vi "Lookup Response Info.vi"(8 "error in (no error)":errorcluster, 9 "Wait Value Channel Lookup Info":T6 {"Refs" format="%.0x"}, 10 "Resp Channel Lookup Info":T6 {"Refs" format="%.0x"}, 11 "Section Ref in":T1 format="%.0x") -> (0 "error out":errorcluster, 1 "Wait Value Channel Lookup Info out":T6 {"Refs" format="%.0x"}, 2 "Resp Channel Lookup Info out":T6 {"Refs" format="%.0x"}, 3 "Section Ref out":T1 format="%.0x", 5 "Response Info":T2)   [LabVIEW 2018, in "Instrument Addon System Explorer.lvlib"]
uses:
  Instrument Addon System Explorer.lvlib
  <vilib>/NI VeriStand/Custom Device Tools/Custom Device Utility Library/Custom Device Utility Library.lvlib
  <vilib>/NI VeriStand/Custom Device Tools/Custom Device Utility Library/NI VeriStand - Search for Item by GUID.vi
  Addon Shared/SubVIs/Constants.vi
  Addon Shared/Instrument Addon Shared.lvlib
  Addon Shared/Types/Response Wait Type.ctl
  Addon Shared/Types/Linked Channel Cluster.ctl
  Addon Shared/Types/Response Parameters.ctl
  Addon Shared/Types/Response RT Configuration Cluster.ctl
  Addon Shared/Types/FG Control.ctl
  <vilib>/NI VeriStand/Custom Device API/Custom Device API.lvlib
  <vilib>/NI VeriStand/Custom Device API/Custom Device Item Ref.ctl
  Types/Channel Lookup Cluster.ctl
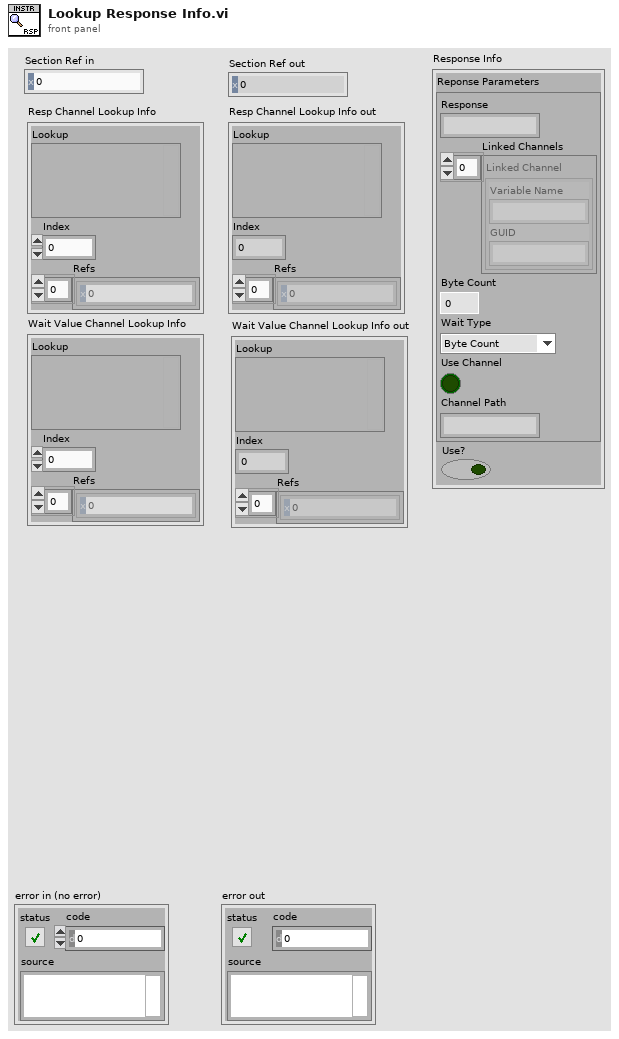
[diagram p1: front panel]
types:
  T1 = typedef "Custom Device API.lvlib/Custom Device Item Ref.ctl" = u64
  T2 = typedef "Instrument Addon Shared.lvlib/Response RT Configuration Cluster.ctl" = cluster{"Reponse Parameters":T3, "Use?":bool}
  T3 = typedef "Instrument Addon Shared.lvlib/Response Parameters.ctl" = cluster{"Response":string, "Linked Channels":T4[], "Type Value":dbl, "Wait Type":T5, "Use Channel":bool, "Channel Path":string}
  T4 = typedef "Instrument Addon Shared.lvlib/Linked Channel Cluster.ctl" = cluster{"Variable Name":string, "GUID":string}
  T5 = typedef "Instrument Addon Shared.lvlib/Response Wait Type.ctl" = enum16{"Byte Count", "Wait sec"}
  T6 = typedef "Instrument Addon System Explorer.lvlib/Channel Lookup Cluster.ctl" = cluster{"Lookup":variant, "Index":i32, "Refs":T1[]}
  T7 = typedef "Instrument Addon Shared.lvlib/FG Control.ctl" = enum16{"Get", "Set"}
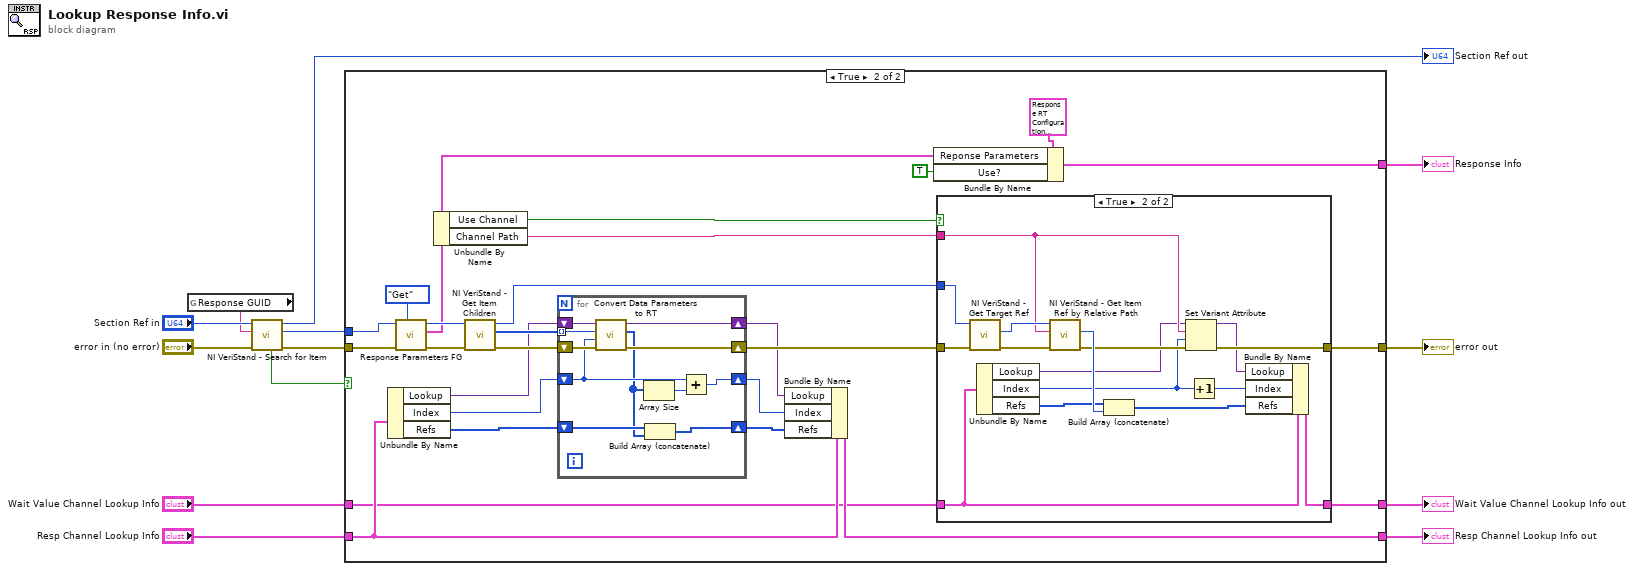
[diagram p0: block diagram]
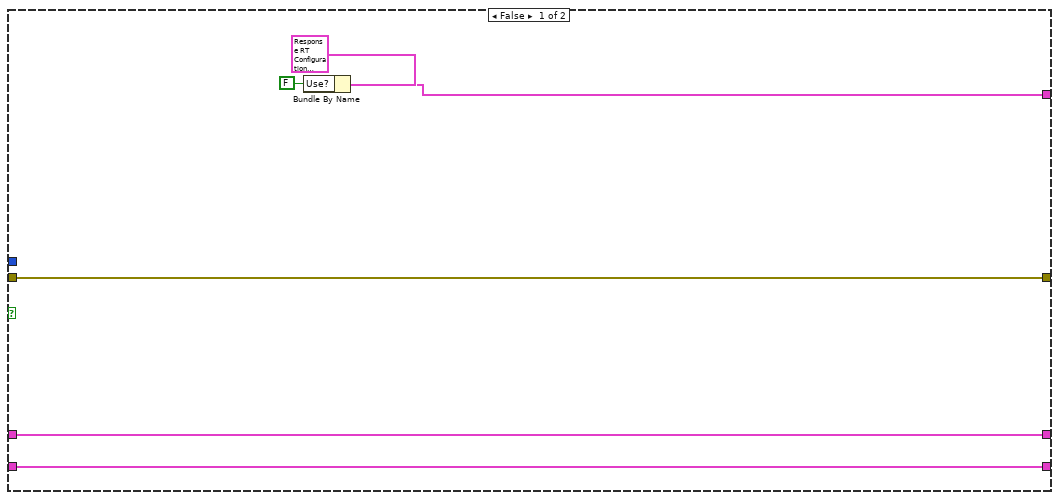
[diagram p2: hidden frame]
diagram:
  n1 = global read "Constants.vi" "Response GUID"() -> (w6:string)
  n2 = call-poly <vilib>:"NI VeriStand - Search for Item.vi"("error in"="error in (no error)", "Item GUID"=w6, "Section Ref in"="Section Ref in") -> ("error out"=w9:errorcluster, "Item Ref"=w10:T1, "Section Ref out"=→"Section Ref out":T1, "Found"=w13:bool)  [unwired: 5 in]
  n3 = case shown="True" w13 {
    tunnel: w9 -> [w19 w44]
    tunnel: w10 -> [_ w43]
    tunnel: [w17 w39] -> w11
    tunnel: [w19 w33] -> w12
    tunnel: "Resp Channel Lookup Info" -> [w15 w27]
    tunnel: [w15 w26] -> w4
    tunnel: "Wait Value Channel Lookup Info" -> [w14 w25]
    tunnel: [w14 w24] -> w2
    frame False {
      n4 = Bundle By Name(cluster=T2 {"Reponse Parameters"={"Response"="", "Linked Channels"=[], "Type Value"=0.0, "Wait Type"=enum."Byte Count", "Use Channel"=FALSE, "Channel Path"=""}, "Use?"=FALSE}, "Use?"=FALSE) -> (w17:T2)
    }
    frame True {
      n5 = Unbundle By Name(w27) -> ("Lookup"=w31:variant, "Index"=w30:i32, "Refs"=w21:T1[])
      n6 = call "Response Parameters FG.vi"("Action"=FG_Control."Get", "error in (no error)"=w44, "Item Ref in"=w43) -> ("error out"=w36:errorcluster, "Reponse Parameters"=w37:T3, "Item Ref out"=w42:T1)  [unwired: 6 in]
      n7 = Unbundle By Name(w37) -> ("Use Channel"=w22:bool, "Channel Path"=w35:string)
      n8 = call <vilib>:"NI VeriStand - Get Item Children.vi"("error in (no error)"=w36, "Item Ref in"=w42) -> ("error out"=w41:errorcluster, "Child Refs"=w38:T1[], "Item Ref out"=w32:T1)  [unwired: 6 in, 1 out]
      n9 = for {
        shift-right: [w71] -> w34
        shift-left: w41 -> [w74]
        tunnel: w38 -> [w73] mode=indexing
        shift-right: [w64] -> w29
        shift-left: w30 -> [w66]
        shift-right: [w70] -> w28
        shift-left: w31 -> [w72]
        shift-right: [w68] -> w20
        shift-left: w21 -> [w69]
        n10 = call "Convert Data Parameters to RT.vi"("error in (no error)"=w74, "Data Index"=w66, "Item Ref in"=w73, "Lookup Table"=w72) -> ("error out"=w71:errorcluster, "Chan Refs"=w65:T1[], "Lookup Table out"=w70:variant)  [unwired: 5 in]
        n11 = Array Size(array=w65) -> (size(s)=w67:i32)
        n12 = Build Array (concatenate)(w69, w65) -> (w68:T1[])
        n13 = Add(x=w66, y=w67) -> (x+y=w64:i32)
      }
      n14 = Bundle By Name(cluster=w27, "Lookup"=w28, "Index"=w29, "Refs"=w20) -> (w26:T6)
      n15 = Bundle By Name(cluster=T2 {"Reponse Parameters"={"Response"="", "Linked Channels"=[], "Type Value"=0.0, "Wait Type"=enum."Byte Count", "Use Channel"=FALSE, "Channel Path"=""}, "Use?"=FALSE}, "Reponse Parameters"=w37, "Use?"=TRUE) -> (w39:T2)
      n16 = case shown="True" w22 {
        tunnel: w35 -> [_ w56]
        tunnel: w34 -> [w47 w61]
        tunnel: [w47 w57] -> w33
        tunnel: w32 -> [_ w60]
        tunnel: w25 -> [w46 w48]
        tunnel: [w46 w49] -> w24
        frame False {
        }
        frame True {
          n17 = call <vilib>:"NI VeriStand - Get Target Ref.vi"("error in"=w61, "Item Ref in"=w60) -> ("error out"=w62:errorcluster, "Target Ref"=w63:T1)  [unwired: 6 in, 2 out]
          n18 = Unbundle By Name(w48) -> ("Lookup"=w55:variant, "Index"=w54:i32, "Refs"=w53:T1[])
          n19 = call <vilib>:"NI VeriStand - Get Item Ref by Relative Path.vi"("error in"=w62, "Relative Item Path"=w56, "Section Ref in"=w63) -> ("error out"=w58:errorcluster, "Item Ref"=w59:T1)  [unwired: 5 in, 2 out]
          n20 = Build Array (concatenate)(w53, w59) -> (w50:T1[])
          n21 = Set Variant Attribute(Variant=w55, name=w56, value=w54, error in=w58) -> (Variant out=w52:variant, error out=w57:errorcluster)  [unwired: 1 out]
          n22 = Increment(x=w54) -> (x+1=w51:i32)
          n23 = Bundle By Name(cluster=w48, "Lookup"=w52, "Index"=w51, "Refs"=w50) -> (w49:T6)
        }
      }
    }
  }
  "Wait Value Channel Lookup Info out" <- w2
  "Resp Channel Lookup Info out" <- w4
  "error out" <- w12
  "Response Info" <- w11
